vi "Proyecto de grado_Aux.vi"() -> ()   [LabVIEW 2025]
panel:
  in  "New Element":i32
  in  "x":i32[](array[numeric])
  out "New list":i32[](array[numeric])
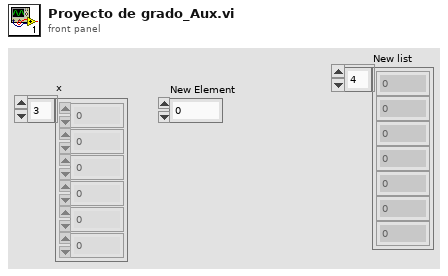
[diagram p1: front panel]
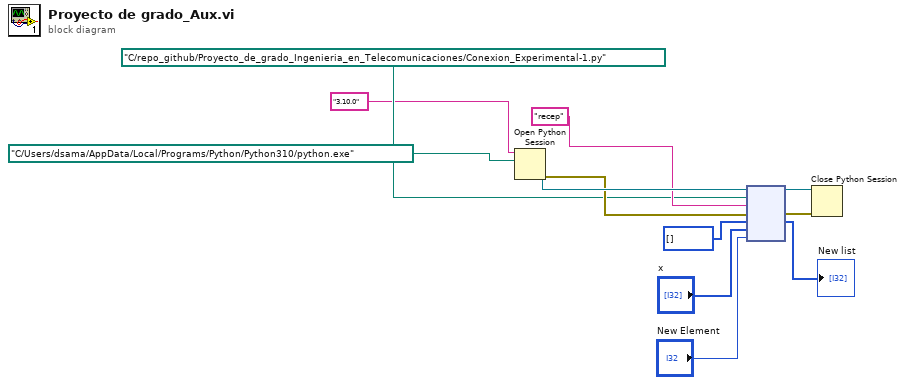
[diagram p0: block diagram]
diagram:
  n1 = Open Python Session(python version="3.10.0" ("Python version"), python path=path "C:/Users/dsama/AppData/Local/Programs/Python/Python310/python.exe" ("Python path")) -> (session out=w12:refnum<k35>, error out=w9:errorcluster)  [unwired: 1 in]
  n2 = node(w12, path "C:/repo_github/Proyecto_de_grado_Ingenieria_en_Telecomunicaciones/Conexion_Experimental-1.py" ("module path"), "recep" ("function name"), w9, i32[] [], "x", "New Element") -> (w11:refnum<k35>, w8:errorcluster, →"New list":i32[])  [unwired: 2 in, 2 out]
  n3 = Close Python Session(session in=w11, error in=w8) -> ()  [unwired: 1 out]
